vi "writeAudio.vi"(8 "error in (no error)":errorcluster, 9 "WAV file reference in":T2, 10 "Trigger timestamps":T3, 11 "Queue in":refnum<queue>) -> (0 "error out":errorcluster, 1 "timeState":T1(ring), 2 "Writing audio?":bool, 3 "WAV file reference out":T2)   [LabVIEW 2017]
doc: "If audio is present in queue, write it to disk."
uses:
  <vilib>/sound2/lvsound2.llb/Sound File Refnum.ctl
  <vilib>/sound2/lvsound2.llb/Sound File Write (DBL).vi
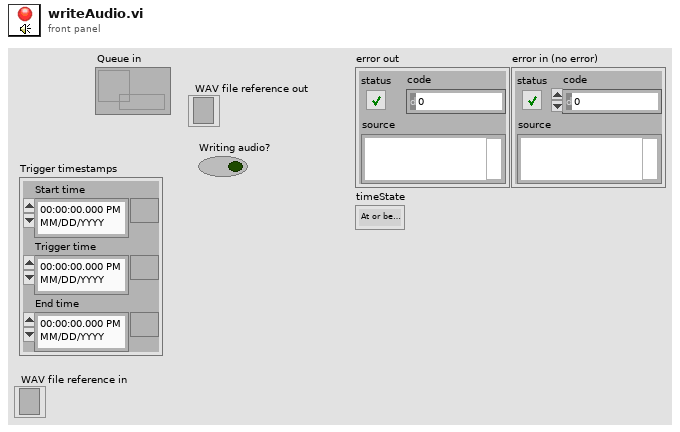
[diagram p1: front panel]
types:
  T1 = enum16{"At or before start", "In range", "At or after end"}
  T2 = typedef "Sound File Refnum.ctl" = refnum<file>
  T3 = cluster{"Start time":timestamp, "Trigger time":timestamp, "End time":timestamp}
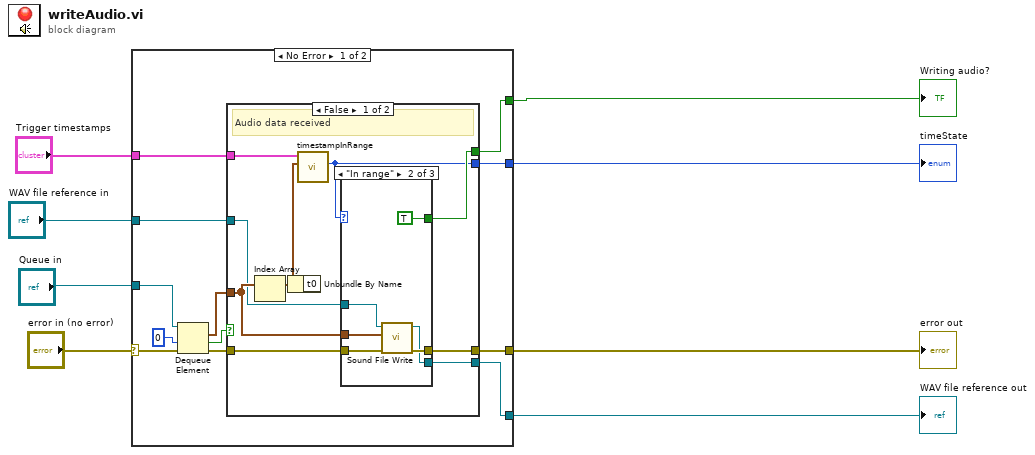
[diagram p0: block diagram]
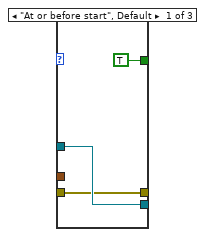
[diagram p2: hidden frame]
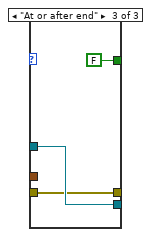
[diagram p3: hidden frame]
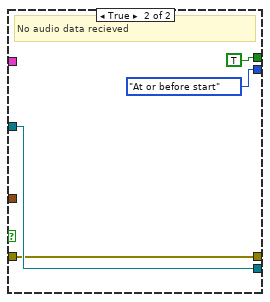
[diagram p4: hidden frame]
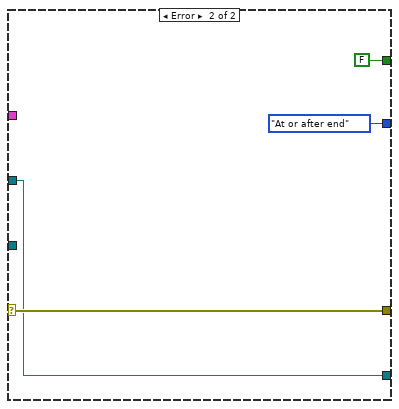
[diagram p5: hidden frame]
diagram:
  n1 = case shown="No Error" "error in (no error)" {
    selector: "error in (no error)" -> [w10 w50]
    tunnel: [w20 FALSE ("Write to file")] -> w8
    tunnel: "Trigger timestamps" -> [w19 _]
    tunnel: [w18 w49] -> w6
    tunnel: "WAV file reference in" -> [w17 w49]
    tunnel: "Queue in" -> [w13 _]
    tunnel: [w11 w50] -> w4
    tunnel: [w9 T1."At or after end" ("timeState")] -> w2
    frame No Error {
      n2 = Dequeue Element(queue=w13, timeout in ms (-1)=0, error in (no error)=w10) -> (element=w15:waveform(dbl)[], timed out?=w14:bool, error out=w16:errorcluster)  [unwired: 1 out]
      n3 = case shown="False" w14 {
        tunnel: w15 -> [w29 _]
        tunnel: w16 -> [w28 w44]
        tunnel: w17 -> [w27 w45]
        tunnel: [w26 TRUE ("Write to file")] -> w20
        tunnel: [w25 w45] -> w18
        tunnel: w19 -> [w24 _]
        tunnel: [w23 w44] -> w11
        tunnel: [w22 T1."At or before start" ("timeState")] -> w9
        frame False {
          # "Audio data received"
          n4 = Index Array(array=w29) -> (element=w21:waveform(dbl))  [unwired: 1 in]
          n5 = Unbundle By Name(w21) -> ("t0"=w30:timestamp)
          n6 = call "timestampInRange.vi"("Time Stamp"=w30, "Start and end times"=w24) -> ("timeState"=w22:T1)  [unwired: 9 in]
          n7 = case shown="\"In range\"" w22 {
            tunnel: w27 -> [w33 w39 w42]
            tunnel: w29 -> [_ w38 _]
            tunnel: w28 -> [w32 w37 w40]
            tunnel: [w32 w36 w40] -> w23
            tunnel: [w33 w35 w42] -> w25
            tunnel: [TRUE ("Write to file") TRUE ("Write to file") FALSE ("Write to file")] -> w26
            frame "At or before start", Default {
            }
            frame "In range" {
              n8 = call-poly <vilib>:"Sound File Write.vi"("error in (no error)"=w37, "data"=w38, "sound file refnum"=w39) -> ("error out"=w36:errorcluster, "sound file refnum out"=w35:T2)  [unwired: 7 in]
            }
            frame "At or after end" {
            }
          }
        }
        frame True {
          # "No audio data recieved"
        }
      }
    }
    frame Error {
    }
  }
  "Writing audio?" <- w8
  "WAV file reference out" <- w6
  "error out" <- w4
  "timeState" <- w2
